vi "System Status.vi"(7 "Box ID":u8, 8 "error in (no error)":errorcluster, 11 "BS120x in":refnum<class "BS120x.lvclass">) -> (0 "error out":errorcluster, 2 "Status":T1, 3 "BS120x out":refnum<class "BS120x.lvclass">)   [LabVIEW 2021, in "BS120x Driver.lvlib" / "BS120x.lvclass"]
doc: "Returns the fan and temperature status of the the Battery Simulator 1200.\n(c) 2019 Bloomy Controls, Inc. All rights reserved."
uses:
  BS120x.lvclass
  TypeDefs/System Status.ctl
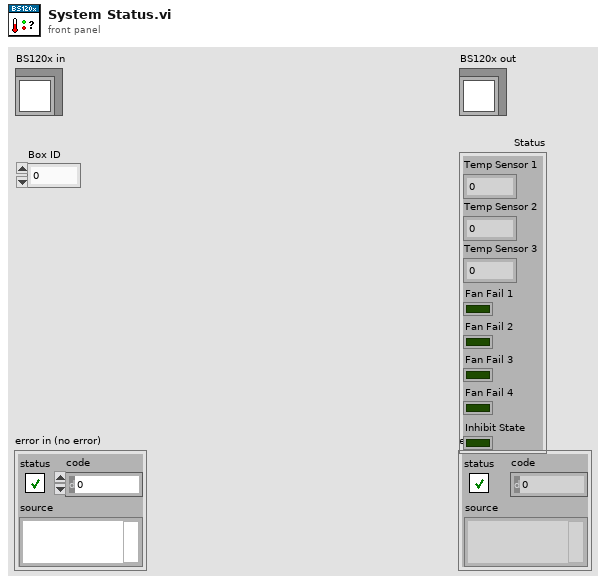
[diagram p1: front panel]
types:
  T1 = typedef "BS120x Driver.lvlib/BS120x.lvclass/System Status.ctl" = cluster{"Temp Sensor 1":dbl, "Temp Sensor 2":dbl, "Temp Sensor 3":dbl, "Fan Fail 1":bool, "Fan Fail 2":bool, "Fan Fail 3":bool, "Fan Fail 4":bool, "Inhibit State":bool}
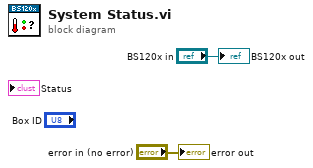
[diagram p0: block diagram]
diagram:
  "error out" <- "error in (no error)"
  "BS120x out" <- "BS120x in"
